vi "calibrationSpectrometerViewMain.vi"(10 "viewThisComponent":refnum<class "ViewThisComponent.lvclass">) -> ()   [LabVIEW 2016]
doc: "Main display method."
uses:
  ComponentTemplateCore/AlarmsTreeDisplay/AlarmsTreeDisplay/Warnings.ctl
  ViewThisComponent/ViewThisComponent.lvclass
  home/harini/tcs/ts_sedspectrometer/ComponentTemplateCore/ComponentModel/ComponentModel/View/View.lvclass
  Settings/ProcessSetting/ProcessSettings.lvclass
  home/harini/tcs/ts_sedspectrometer/Settings/Settings/Setting.lvclass
  Settings/SettingsTC/TCSettings.lvclass
  View/AlarmsTreeDisplayTC/AlarmsTreeDisplayTC.lvclass
  <vilib>/Utility/error.llb/DialogType.ctl
  ts_sallv_sedspectrometer/DataTypes/logevent_SummaryState.ctl
  Settings/Settings/Setting.lvclass/Setting.ctl
  <vilib>/Platform/browser.llb/Open URL in Default Browser (string).vi
  ComponentTemplateCore/AlarmsTreeDisplay/AlarmsTreeDisplay/AlarmsTreeDisplay.lvclass
  View/ViewElements/calibrationSpectrometerViewElements.lvlib
  ComponentTemplateCore/ComponentModel/ComponentModel/View/View.lvclass
  ComponentTemplateCore/Internet/Internet.lvclass
  Settings/Settings/Setting.lvclass
  ComponentTemplateCore/ComponentModel/ComponentModel/ConfigurationFileReader/ConfigurationFileReader.lvclass
  ts_sallv_sedspectrometer/SALLV_calibrationSpectrometer.lvlib
panel:
  in  "Settings This Component":refnum<class "TCSettings.lvclass">
  in  "Common Settings":refnum<class "ProcessSettings.lvclass">
  out "Warnings Tree":T1 caption="Warnings"
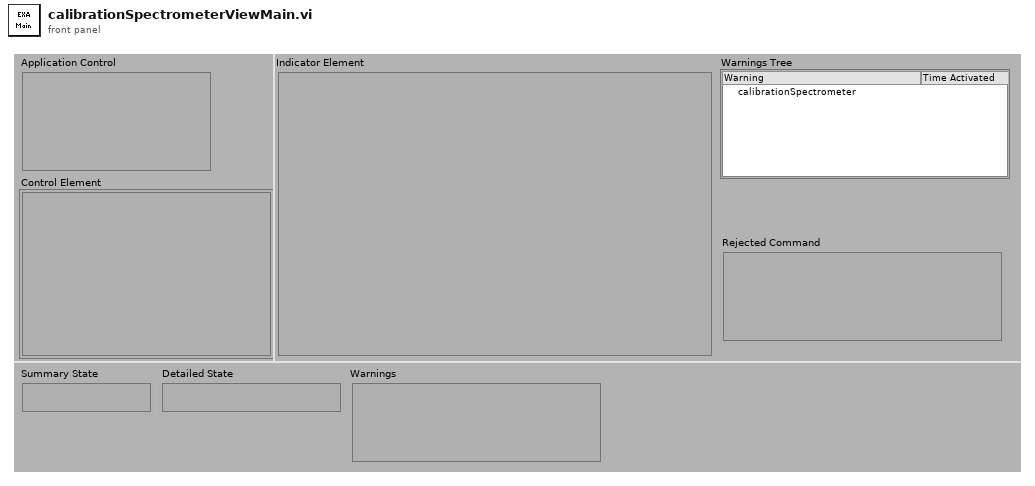
[diagram p1: front panel]
types:
  T1 = typedef "AlarmsTreeDisplay.lvclass/Warnings.ctl" = string
  T2 = typedef "TypedefsDataEvents.lvlib/PubDataEvents.ctl" = cluster{"AppliedSettingsMatchStart":refnum<user-event>, "SettingVersions":refnum<user-event>, "SummaryState":refnum<user-event>, "RejectedCommand":refnum<user-event>, "DetailedState":refnum<user-event>, "ErrorCode":refnum<user-event>, "Heartbeat":refnum<user-event>, "LoopTime_ms":refnum<user-event>, "LoopTimeOutOfRange":refnum<user-event>, "Timestamp":refnum<user-event>, "TimeOut":refnum<user-event>, "MeasuredSpectrum":refnum<user-event>}
  T3 = typedef "SALLV_calibrationSpectrometer.lvlib/logevent_SummaryState.ctl" = cluster{"summaryState":enum16{"", "DisabledState", "EnabledState", "FaultState", "OfflineState", "StandbyState"}, "priority":i32}
  T4 = typedef "DialogType.ctl" = u16
  T5 = enum16{"", "DisabledState", "EnabledState", "FaultState", "OfflineState", "StandbyState"}
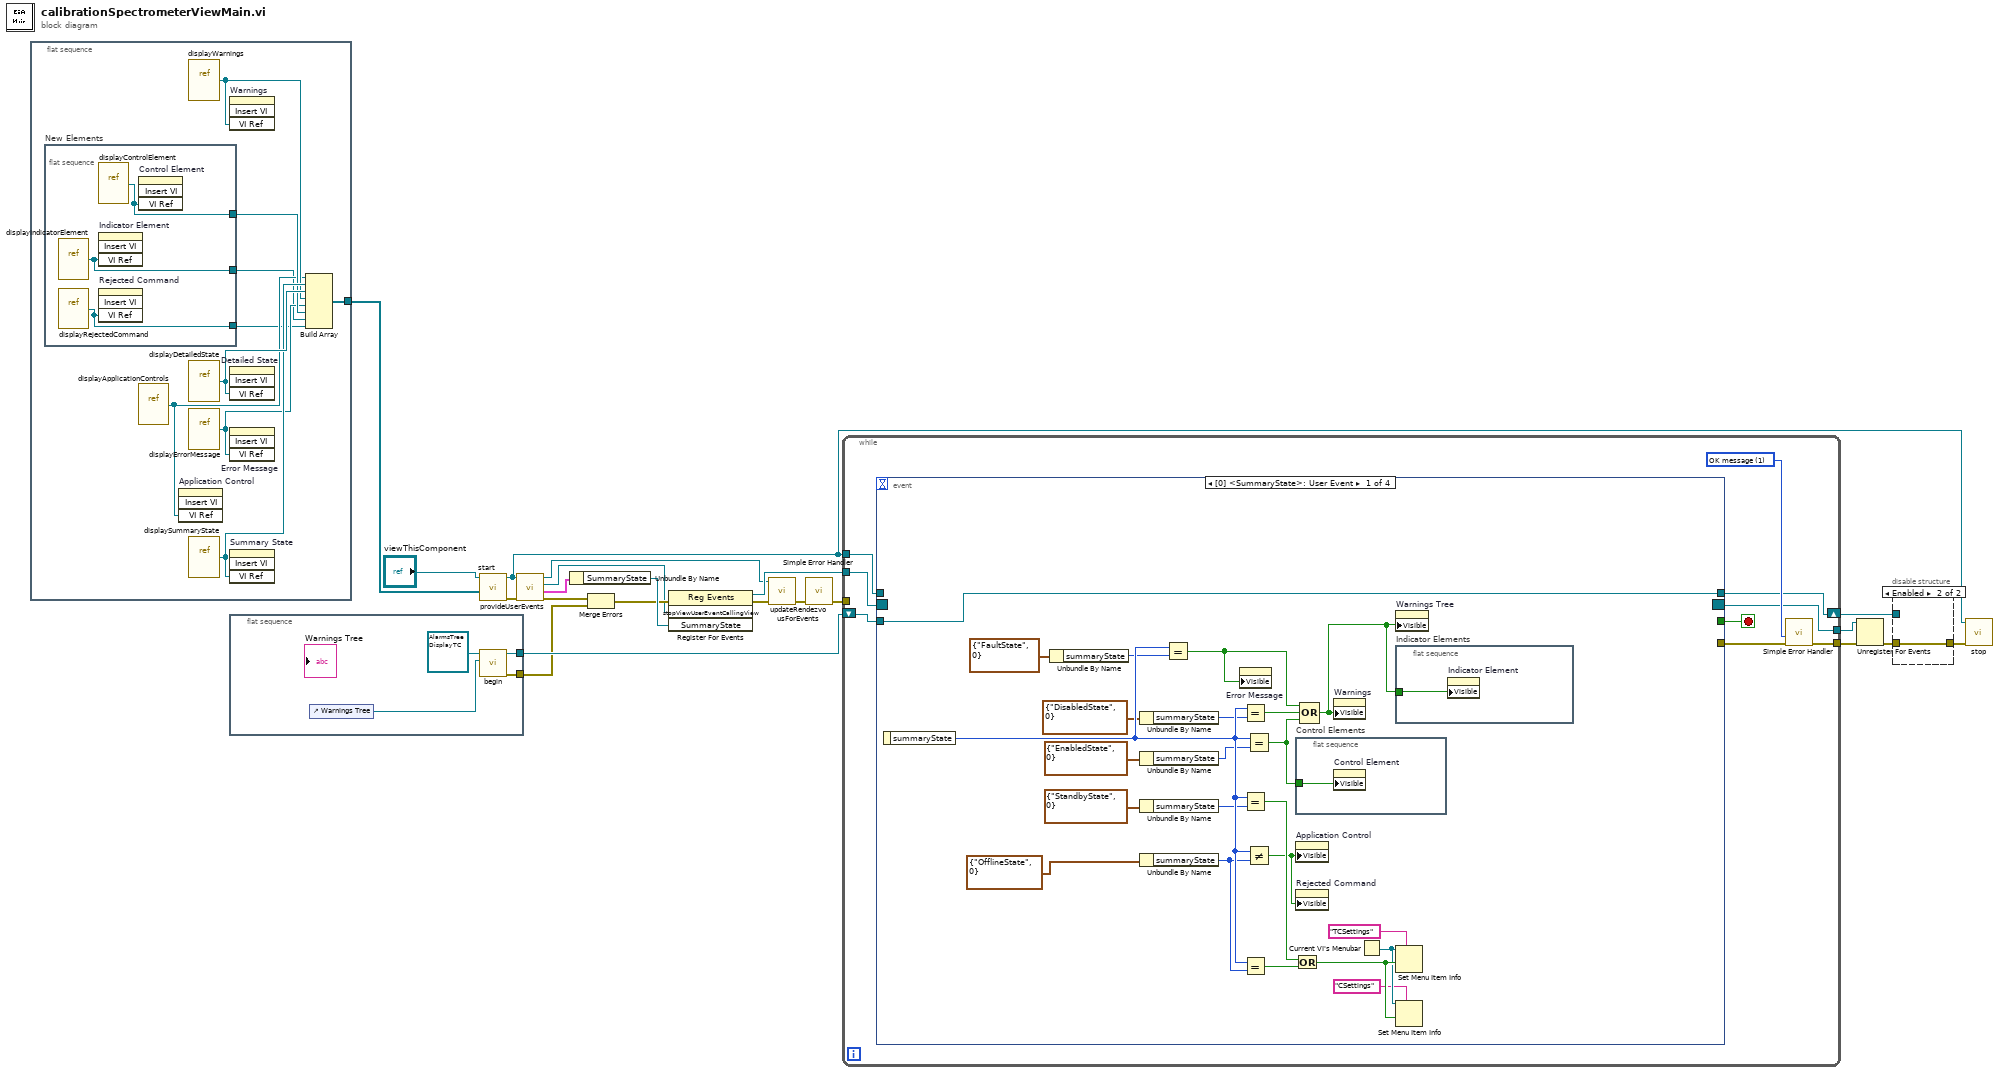
[diagram p0: block diagram]
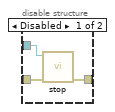
[diagram p2: hidden frame]
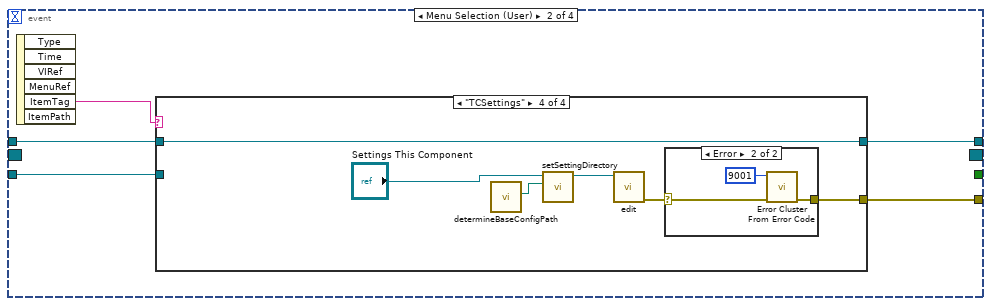
[diagram p3: hidden frame]
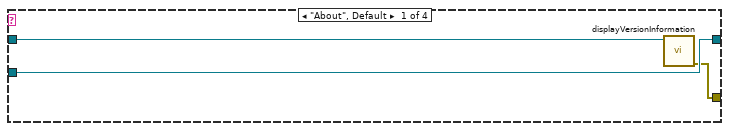
[diagram p4: hidden frame]
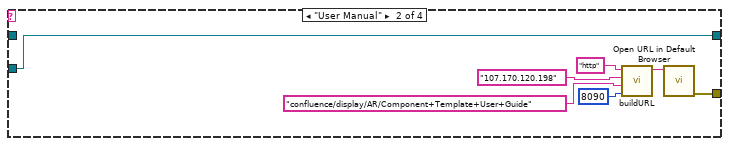
[diagram p5: hidden frame]
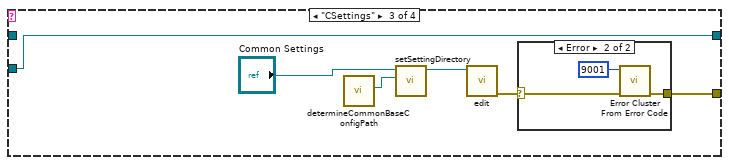
[diagram p6: hidden frame]
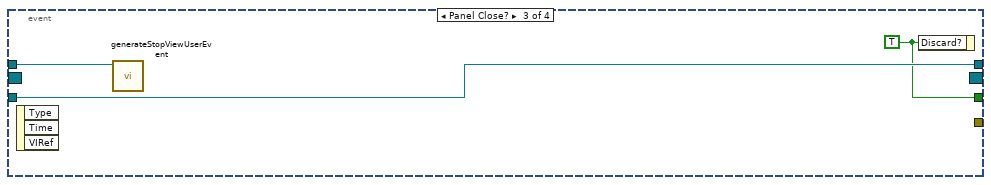
[diagram p9: hidden frame]
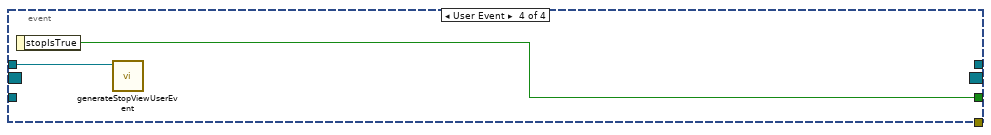
[diagram p10: hidden frame]
diagram:
  n1 = flat-sequence {
    tunnel: [w28] -> w17
    frame #0 {
      n2 = flat-sequence "New Elements" {
        tunnel: [w33] -> w26
        tunnel: [w32] -> w23
        tunnel: [w31] -> w22
        frame #0 {
          n3 = vi-ref "displayIndicatorElement.vi"() -> (w32:refnum<vi>)
          n4 = vi-ref "displayRejectedCommand.vi"() -> (w31:refnum<vi>)
          n5 = vi-ref "displayControlElement.vi"() -> (w33:refnum<vi>)
          n6 = invoke on="Indicator Element" class="SubPanel" method="Insert VI"("VI Ref"=w32) -> ()  [unwired: 3 in, 4 out]
          n7 = invoke on="Rejected Command" class="SubPnl" method="Insert VI"("VI Ref"=w31) -> ()  [unwired: 3 in, 4 out]
          n8 = invoke on="Control Element" class="SubPnl" method="Insert VI"("VI Ref"=w33) -> ()  [unwired: 3 in, 4 out]
        }
      }
      n9 = vi-ref "displayApplicationControls.vi"() -> (w25:refnum<vi>)
      n10 = invoke on="Application Control" class="SubPanel" method="Insert VI"("VI Ref"=w25) -> ()  [unwired: 3 in, 4 out]
      n11 = vi-ref "displayWarnings.vi"() -> (w27:refnum<vi>)
      n12 = vi-ref "displayDetailedState.vi"() -> (w30:refnum<vi>)
      n13 = vi-ref "displayErrorMessage.vi"() -> (w24:refnum<vi>)
      n14 = vi-ref "displaySummaryState.vi"() -> (w29:refnum<vi>)
      n15 = invoke on="Warnings" class="SubPanel" method="Insert VI"("VI Ref"=w27) -> ()  [unwired: 3 in, 4 out]
      n16 = invoke on="Detailed State" class="SubPanel" method="Insert VI"("VI Ref"=w30) -> ()  [unwired: 3 in, 4 out]
      n17 = invoke on="Error Message" class="SubPanel" method="Insert VI"("VI Ref"=w24) -> ()  [unwired: 3 in, 4 out]
      n18 = invoke on="Summary State" class="SubPanel" method="Insert VI"("VI Ref"=w29) -> ()  [unwired: 3 in, 4 out]
      n19 = Build Array(w25, w29, w30, w27, w24, w26, w23, w22) -> (w28:refnum<vi>[])
    }
  }
  n20 = flat-sequence {
    tunnel: [w34] -> w21
    tunnel: [w35] -> w18
    frame #0 {
      n21 = control-ref of="Warnings Tree"() -> (w37:refnum<vi>)
      n22 = call "begin.vi"("alarmTreeRefnum"=w37, "AlarmsTreeDisplayTC in"=refnum<class "AlarmsTreeDisplayTC.lvclass"> refnum) -> ("error out"=w35:errorcluster, "AlarmsTreeDisplayTC out"=w34:refnum<class "AlarmsTreeDisplayTC.lvclass">)  [unwired: 8 in]
    }
  }
  n23 = call-dynamic "start.vi"("subpanelVIRefs"=w17, "View in"="viewThisComponent") -> ("error out"=w5:errorcluster, "View out"=w8:refnum<class "ViewThisComponent.lvclass">)  [unwired: 8 in]
  n24 = call "provideUserEvents.vi"("error in (no error)"=w5, "ViewThisComponent in"=w8) -> ("error out"=w4:errorcluster, "pubDataEvents"=w6:T2, "stopViewUserEventCallingView"=w7:refnum<user-event>, "ViewThisComponent out"=w1:refnum<class "ViewThisComponent.lvclass">)  [unwired: 6 in]
  n25 = Unbundle By Name(w6) -> ("SummaryState"=w16:refnum<user-event>)
  n26 = Merge Errors(w4, w18) -> (w14:errorcluster)
  n27 = register-events(error in=w14, w7, w16) -> (reference out=w15:refnum<event-registration>, error out=w3:errorcluster)  [unwired: 1 in]
  n28 = call "updateRendezvousForEvents.vi"("error in (no error)"=w3, "View in"=w1) -> ("error out"=w2:errorcluster)  [unwired: 8 in, 1 out]
  n29 = call <vilib>:"Simple Error Handler.vi"("error in (no error)"=w2) -> ("error out"=w19:errorcluster)  [unwired: 4 in, 4 out]
  n30 = while {
    tunnel: w15 -> [w46]
    shift-right: [w43] -> w20
    shift-left: w21 -> [w44]
    tunnel: w19 -> [_]
    tunnel: w8 -> [w41]
    tunnel: [w39] -> w12
    tunnel: [w38] -> w13
    stop <- w42 stop-if-true
    w45 = T4 1 items=["no dialog", "OK message", "continue or stop message", "OK message + warnings", "continue/stop + warnings"] ("type of dialog (OK msg:1)")
    n31 = event shown="[0] <SummaryState>: User Event" {
      selector: w46 -> [_ _ _ _]
      dyn-events: [_ _ _ _] -> w38
      timeout: _ -> [_ _ _ _]
      tunnel: [_ w75 _ _] -> w40
      tunnel: w44 -> [w69 w74 w109 _]
      tunnel: [w69 w73 w109 _] -> w43
      tunnel: [_ _ w108 w111] -> w42
      tunnel: w41 -> [_ w72 w107 w110]
      event User Event {
        n32 = event-data() -> ("summaryState"=w68:T5)  [unwired: 1 in]
        n33 = Unbundle By Name(T3 {"summaryState"=enum."FaultState", "priority"=0} ("logevent_SummaryState")) -> ("summaryState"=w51:T5)
        n34 = Unbundle By Name(T3 {"summaryState"=enum."DisabledState", "priority"=0} ("logevent_SummaryState")) -> ("summaryState"=w55:T5)
        n35 = Unbundle By Name(T3 {"summaryState"=enum."EnabledState", "priority"=0} ("logevent_SummaryState")) -> ("summaryState"=w53:T5)
        n36 = Unbundle By Name(T3 {"summaryState"=enum."StandbyState", "priority"=0} ("logevent_SummaryState")) -> ("summaryState"=w49:T5)
        n37 = Unbundle By Name(T3 {"summaryState"=enum."OfflineState", "priority"=0} ("logevent_SummaryState")) -> ("summaryState"=w48:T5)
        n38 = Equal?(x=w68, y=w51) -> (x = y?=w62:bool)
        n39 = property on="Error Message" class="SubPnl"("Visible"=w62) -> ()  [unwired: 2 in, 2 out]
        n40 = Equal?(x=w68, y=w55) -> (x = y?=w64:bool)
        n41 = Equal?(x=w68, y=w49) -> (x = y?=w65:bool)
        n42 = Equal?(x=w68, y=w48) -> (x = y?=w66:bool)
        n43 = Equal?(x=w68, y=w53) -> (x = y?=w63:bool)
        n44 = Not Equal?(x=w68, y=w48) -> (x != y?=w60:bool)
        n45 = Or(x=w65, y=w66) -> (x .or. y?=w59:bool)
        n46 = flat-sequence "Control Elements" {
          tunnel: w63 -> [w70]
          frame #0 {
            n47 = property on="Control Element" class="SubPnl"("Visible"=w70) -> ()  [unwired: 2 in, 2 out]
          }
        }
        n48 = property on="Application Control" class="SubPnl"("Visible"=w60) -> ()  [unwired: 2 in, 2 out]
        n49 = property on="Rejected Command" class="SubPnl"("Visible"=w60) -> ()  [unwired: 2 in, 2 out]
        n50 = Compound Arithmetic op=OR(w62, w64, w63) -> (w61:bool)
        n51 = property on="Warnings" class="SubPnl"("Visible"=w61) -> ()  [unwired: 2 in, 2 out]
        n52 = Current VI's Menubar() -> (w58:refnum<k9>)
        n53 = property on="Warnings Tree" class="Tree (strict)"("Visible"=w61) -> ()  [unwired: 2 in, 2 out]
        n54 = flat-sequence "Indicator Elements" {
          tunnel: w61 -> [w71]
          frame #0 {
            n55 = property on="Indicator Element" class="SubPnl"("Visible"=w71) -> ()  [unwired: 2 in, 2 out]
          }
        }
        n56 = Set Menu Item Info(7:"TCSettings" ("item name"), 9:w59, 11:w58) -> ()  [unwired: 4 in, 2 out]
        n57 = Set Menu Item Info(7:"CSettings" ("item name"), 9:w59, 11:w58) -> ()  [unwired: 4 in, 2 out]
      }
      event Menu Selection (User) {
        n58 = event-data() -> ("ItemTag"=w76:string)  [unwired: 1 in, 5 out]
        n59 = case shown="\"TCSettings\"" w76 {
          tunnel: [w78 w82 w87 w97] -> w75
          tunnel: w74 -> [w79 w86 w92 _]
          tunnel: [w79 w86 w92 w101] -> w73
          tunnel: w72 -> [w77 _ _ w101]
          frame "About", Default {
            n60 = call-dynamic "displayVersionInformation.vi"("View in"=w77) -> ("error out"=w78:errorcluster)  [unwired: 9 in, 1 out]
          }
          frame "User Manual" {
            n61 = call "buildURL.vi"("port (default)"=8090, "virtual path (none)"="confluence/display/AR/Component+Template+User+Guide", "host (this computer)"="107.170.120.198", "protocol (http)"="http") -> ("url"=w84:string)  [unwired: 7 in]
            n62 = call-poly <vilib>:"Open URL in Default Browser.vi"("URL"=w84) -> ("error out"=w82:errorcluster)  [unwired: 5 in, 1 out]
          }
          frame "CSettings" {
            n63 = call "determineCommonBaseConfigPath.vi"() -> ("ConfigurationPath"=w89:path)  [unwired: 9 in, 2 out]
            n64 = call "setSettingDirectory.vi"("SettingDirectory"=w89, "BaseSetting in"="Common Settings") -> ("BaseSetting out"=w90:refnum<class "ProcessSettings.lvclass">)  [unwired: 9 in]
            n65 = call-dynamic "edit.vi"("BaseSetting in"=w90) -> ("error out"=w88:errorcluster)  [unwired: 8 in, 2 out]
            n66 = case shown="Error" w88 {
              selector: w88 -> [w93 w96]
              tunnel: [w93 w95] -> w87
              frame No Error {
              }
              frame Error {
                n67 = call <vilib>:"Error Cluster From Error Code.vi"("error in (no error)"=w96, "error code (0)"=9001) -> ("error out"=w95:errorcluster)  [unwired: 7 in]
              }
            }
          }
          frame "TCSettings" {
            n68 = call "determineBaseConfigPath.vi"() -> ("baseConfigPath"=w99:path)  [unwired: 9 in, 2 out]
            n69 = call "setSettingDirectory.vi"("SettingDirectory"=w99, "BaseSetting in"="Settings This Component") -> ("BaseSetting out"=w102:refnum<class "TCSettings.lvclass">)  [unwired: 9 in]
            n70 = call-dynamic "edit.vi"("TCSettings in"=w102) -> ("error out"=w98:errorcluster)  [unwired: 8 in, 2 out]
            n71 = case shown="Error" w98 {
              selector: w98 -> [w103 w106]
              tunnel: [w103 w105] -> w97
              frame No Error {
              }
              frame Error {
                n72 = call <vilib>:"Error Cluster From Error Code.vi"("error in (no error)"=w106, "error code (0)"=9001) -> ("error out"=w105:errorcluster)  [unwired: 7 in]
              }
            }
          }
        }
      }
      event Panel Close? {
        w108 = TRUE ("Discard?")
        n73 = event-data() -> ()  [unwired: 1 in, 3 out]
        n74 = call "generateStopViewUserEvent.vi"("View in"=w107) -> ()  [unwired: 9 in, 2 out]
        n75 = event-data("Discard?"=w108) -> ()  [unwired: 1 in, 1 out]
      }
      event User Event {
        n76 = event-data() -> ("stopIsTrue"=w111:bool)  [unwired: 1 in]
        n77 = call "generateStopViewUserEvent.vi"("View in"=w110) -> ()  [unwired: 9 in, 2 out]
      }
    }
    n78 = call <vilib>:"Simple Error Handler.vi"("type of dialog (OK msg:1)"=w45, "error in (no error)"=w40) -> ("error out"=w39:errorcluster)  [unwired: 3 in, 4 out]
  }
  n79 = Unregister For Events(event registration refnum=w13, error in=w12) -> (error out=w11:errorcluster)
  n80 = disable-structure shown="Enabled" {
    disable-tunnel: w20 -> [w114 _]
    disable-tunnel: w11 -> [w113 w115]
    disable-tunnel: [w112 w115] -> w9
    frame Disabled {
      n81 = call "stop.vi"("error in (no error)"=w113, "AlarmsTreeDisplay in"=w114) -> ("error out"=w112:errorcluster)  [unwired: 8 in, 1 out]
    }
    frame Enabled {
    }
  }
  n82 = call-dynamic "stop.vi"("error in (no error)"=w9, "View in"=w8) -> ()  [unwired: 8 in, 2 out]
